vi "Handle Depth Image.vi"(4 "queue in":refnum<queue>, 5 "Event Data":cluster{"sender":refnum<k24>, "e":refnum<k24>}, 6 "Control Ref":refnum<k24>, 7 "Event Common Data":T1) -> ()   [LabVIEW 2011]
uses:
  <vilib>/vision/Image Controls.llb/IMAQ Image.ctl
  Microsoft.Research.Kinect
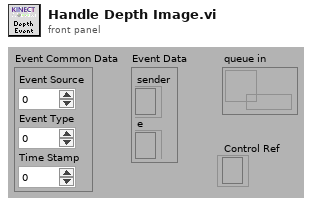
[diagram p1: front panel]
types:
  T1 = cluster{"Event Source":i32, "Event Type":u32, "Time Stamp":u32}
  T2 = typedef "Image Type" = u32
  T3 = typedef "IMAQ Image.ctl" = refnum<image>
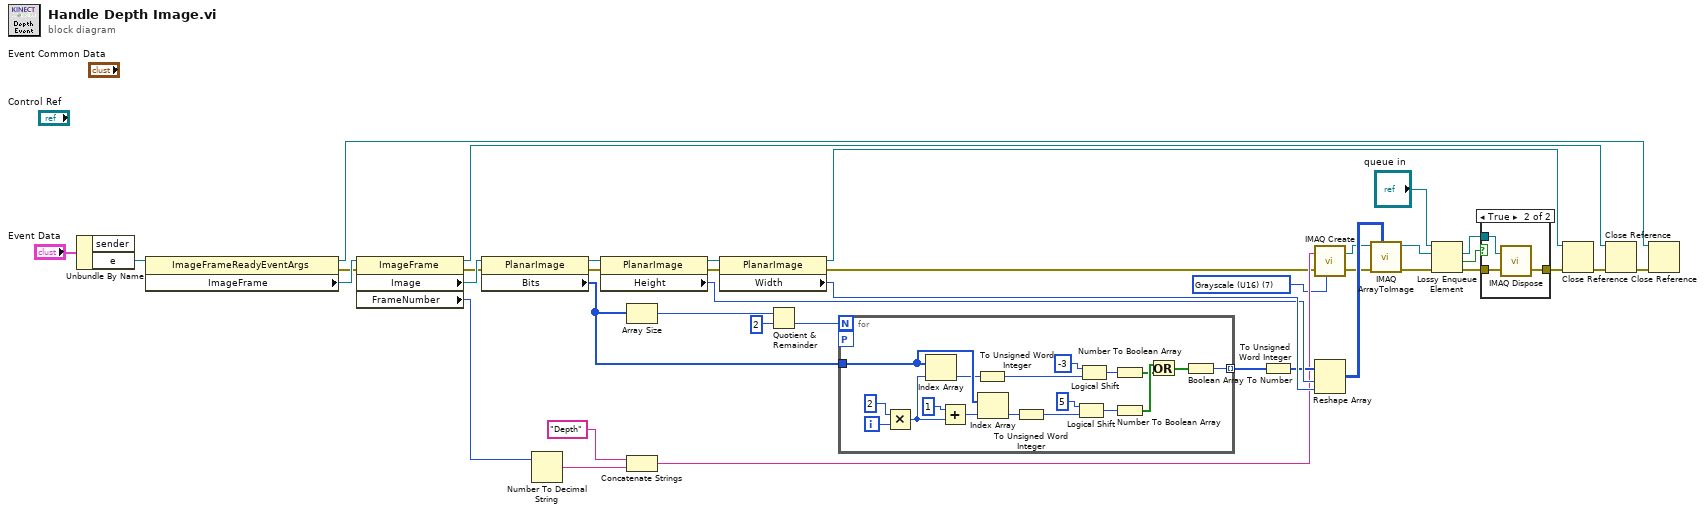
[diagram p0: block diagram]
diagram:
  w7 = T2 7 items=["Grayscale (U8)", "Grayscale (I16)", "Grayscale (SGL)", "Complex (CSG)", "RGB (U32)", "HSL (U32)", "RGB (U64)", "Grayscale (U16)"] ("Image Type")
  n1 = Unbundle By Name("Event Data") -> ("e"=w39:refnum<k24>)  [unwired: 1 out]
  n2 = property class="ImageFrameReadyEventArgs"(reference=w39) -> (reference out=w21:refnum<k24>, error out=w18:errorcluster, "ImageFrame"=w38:refnum<k24>)  [unwired: 1 in]
  n3 = property class="ImageFrame"(reference=w38, error in=w18) -> (reference out=w22:refnum<k24>, error out=w19:errorcluster, "Image"=w26:refnum<k24>, "FrameNumber"=w15:i32)
  n4 = property class="PlanarImage"(reference=w26, error in=w19) -> (reference out=w35:refnum<k24>, error out=w37:errorcluster, "Bits"=w34:u8[])
  n5 = Number To Decimal String(number=w15) -> (decimal integer string=w10:string)  [unwired: 1 in]
  n6 = property class="PlanarImage"(reference=w35, error in=w37) -> (reference out=w29:refnum<k24>, error out=w36:errorcluster, "Height"=w27:i32)
  n7 = Array Size(array=w34) -> (size(s)=w33:i32)
  n8 = Concatenate Strings("Depth" ("string"), w10) -> (w8:string)
  n9 = property class="PlanarImage"(reference=w29, error in=w36) -> (reference out=w30:refnum<k24>, error out=w5:errorcluster, "Width"=w28:i32)
  n10 = Quotient & Remainder(x=w33, y=2) -> (floor(x/y)=w31:i32)  [unwired: 1 out]
  n11 = for {
    N: w31 -> [_]
    tunnel: w34 -> [w52]
    tunnel: [w46] -> w17 mode=indexing
    workers-P: _ -> [_]
    i -> [w49]
    n12 = Multiply(x=2, y=w49) -> (x*y=w47:i32)
    n13 = Index Array(array=w52, index=w47) -> (element=w45:u8)
    n14 = Add(x=1, y=w47) -> (x+y=w50:i32)
    n15 = To Unsigned Word Integer(number=w45) -> (unsigned 16bit integer=w42:u16)
    n16 = Index Array(array=w52, index=w50) -> (element=w44:u8)
    n17 = To Unsigned Word Integer(number=w44) -> (unsigned 16bit integer=w43:u16)
    n18 = Logical Shift(y=5, x=w43) -> (x << y=w57:u16)
    n19 = Logical Shift(y=-3, x=w42) -> (x << y=w56:u16)
    n20 = Number To Boolean Array(number=w56) -> (Boolean array=w54:bool[])
    n21 = Number To Boolean Array(number=w57) -> (Boolean array=w55:bool[])
    n22 = Or(x=w55, y=w54) -> (x .or. y?=w53:bool[])
    n23 = Boolean Array To Number(Boolean array=w53) -> (number=w46:u32)
  }
  n24 = To Unsigned Word Integer(number=w17) -> (unsigned 16bit integer=w16:u16[])
  n25 = call "IMAQ Create"("Image Name"=w8, "Image Type"=w7, "error in (no error)"=w5) -> ("New Image"=w14:T3, "error out"=w13:errorcluster)  [unwired: 2 in]
  n26 = Reshape Array(w16, w27, w28) -> (w25:u16[][])
  n27 = call "IMAQ ArrayToImage"("Image Pixels (U16)"=w25, "error in (no error)"=w13, "Image"=w14) -> ("error out"=w12:errorcluster, "Image Out"=w11:T3)  [unwired: 7 in]
  n28 = Lossy Enqueue Element(queue="queue in", element=w11, error in (no error)=w12) -> (overflow element=w4:T3, overflow?=w1:bool, error out=w3:errorcluster)  [unwired: 1 out]
  n29 = case shown="True" w1 {
    tunnel: w4 -> [_ w61]
    tunnel: w3 -> [w58 w60]
    tunnel: [w58 w59] -> w2
    frame False {
    }
    frame True {
      n30 = call "IMAQ Dispose"("Image"=w61, "error in (no error)"=w60) -> ("error out"=w59:errorcluster)  [unwired: 4 in]
    }
  }
  n31 = Close Reference(reference=w30, error in (no error)=w2) -> (error out=w24:errorcluster)
  n32 = Close Reference(reference=w22, error in (no error)=w24) -> (error out=w23:errorcluster)
  n33 = Close Reference(reference=w21, error in (no error)=w23) -> ()  [unwired: 1 out]
